vi "Speed from Pulse Position (No State).vi"(6 "state in":T1, 7 "Blocks/Pulse":dbl, 10 "pulse/revolution (1)":dbl, 11 "speed position info":T2) -> (3 "CPS":dbl, 4 "state out":T1)   [LabVIEW 2012, in "Measurement Channels.lvlib" / "Tachometer.lvclass"]
uses:
  Tachometer.lvclass
  <vilib>/addons/Sound and Vibration/Order Analysis/Misc/OAT Position Info.ctl
  <vilib>/Analysis/baseanly.llb/Mean (DBL).vi
  <vilib>/Analysis/NI_AALBase.lvlib
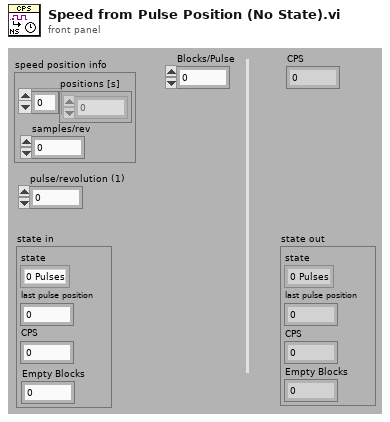
[diagram p1: front panel]
types:
  T1 = cluster{"state":enum16{"0 Pulses", "1 Pulse", "2+ Pulses"}, "last pulse position":dbl, "CPS":dbl, "Empty Blocks":i32}
  T2 = typedef "OAT Position Info.ctl" = cluster{"positions [s]":dbl[], "samples/rev":dbl}
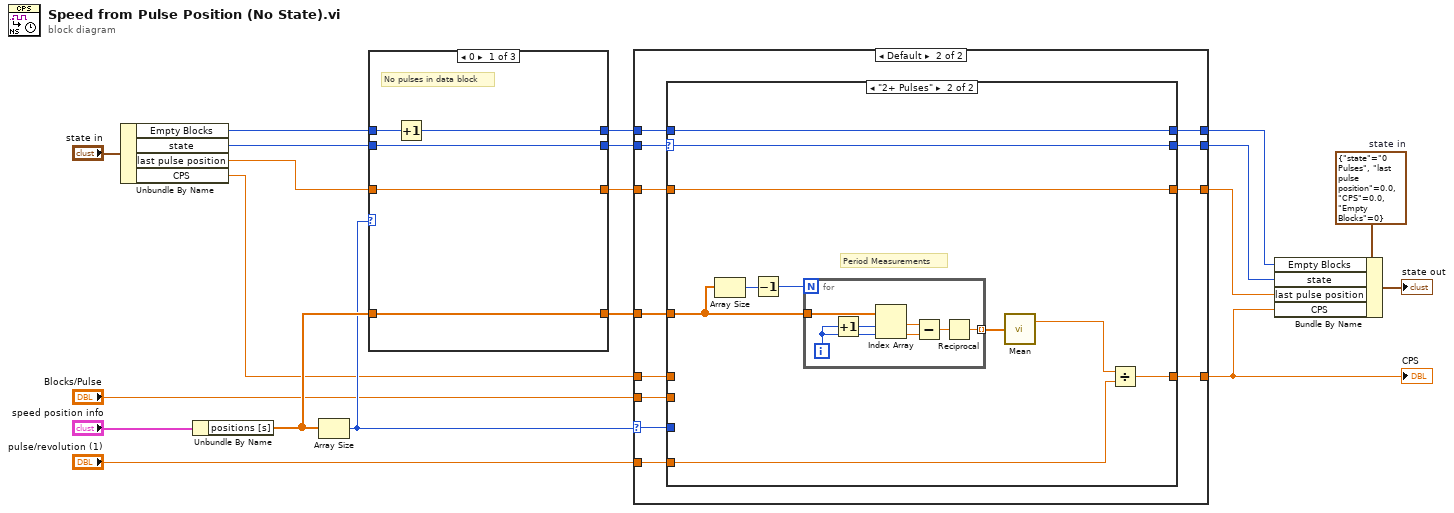
[diagram p0: block diagram]
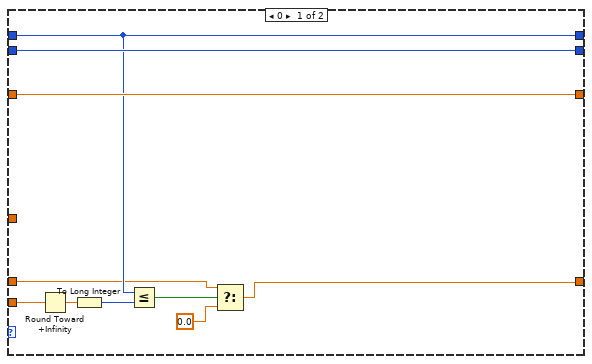
[diagram p2: hidden frame]
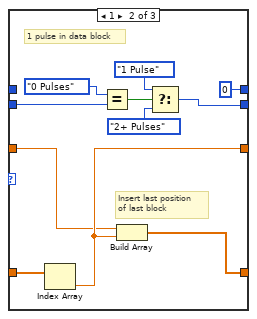
[diagram p4: hidden frame]
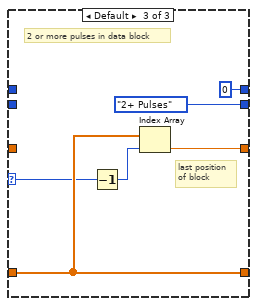
[diagram p5: hidden frame]
diagram:
  w6 = T1 {"state"=enum."0 Pulses", "last pulse position"=0.0, "CPS"=0.0, "Empty Blocks"=0}  # state in
  n1 = Unbundle By Name("state in") -> ("Empty Blocks"=w4:i32, "state"=w9:enum16{"0 Pulses", "1 Pulse", "2+ Pulses"}, "last pulse position"=w8:dbl, "CPS"=w7:dbl)
  n2 = Unbundle By Name("speed position info") -> ("positions [s]"=w16:dbl[])
  n3 = Array Size(array=w16) -> (size(s)=w14:i32)
  n4 = case shown="0" w14 {
    selector: w14 -> [_ _ w41]
    tunnel: w8 -> [w24 w33 _]
    tunnel: [w24 w34 w39] -> w13
    tunnel: w9 -> [w25 w31 _]
    tunnel: [w25 w27 enum16{"0 Pulses", "1 Pulse", "2+ Pulses"}."2+ Pulses" ("Enum")] -> w11
    tunnel: w16 -> [w23 w36 w42]
    tunnel: [w23 w35 w42] -> w10
    tunnel: w4 -> [w22 _ _]
    tunnel: [w21 0 0] -> w3
    frame 0 {
      # "No pulses in data block"
      n5 = Increment(x=w22) -> (x+1=w21:i32)
    }
    frame 1 {
      # "Insert last position\nof last block"
      # "1 pulse in data block"
      n6 = Index Array(array=w36) -> (element=w34:dbl)  [unwired: 1 in]
      n7 = Equal?(x=enum16{"0 Pulses", "1 Pulse", "2+ Pulses"}."0 Pulses" ("Enum"), y=w31) -> (x = y?=w30:bool)
      n8 = Build Array(w33, w34) -> (w35:dbl[])
      n9 = Select(t=enum16{"0 Pulses", "1 Pulse", "2+ Pulses"}."1 Pulse" ("Enum"), s=w30, f=enum16{"0 Pulses", "1 Pulse", "2+ Pulses"}."2+ Pulses" ("Enum")) -> (s? t:f=w27:enum16{"0 Pulses", "1 Pulse", "2+ Pulses"})
    }
    frame Default {
      # "last position\nof block"
      # "2 or more pulses in data block"
      n10 = Decrement(x=w41) -> (x-1=w40:i32)
      n11 = Index Array(array=w42, index=w40) -> (element=w39:dbl)
    }
  }
  n12 = case shown="Default" w14 {
    selector: w14 -> [_ w56]
    tunnel: w10 -> [_ w64]
    tunnel: w11 -> [w52 w63]
    tunnel: [w43 w62] -> w20
    tunnel: w7 -> [w44 w61]
    tunnel: "pulse/revolution (1)" -> [_ w60]
    tunnel: [w52 w59] -> w17
    tunnel: w13 -> [w51 w58]
    tunnel: [w51 w57] -> w18
    tunnel: w3 -> [w45 w55]
    tunnel: [w45 w54] -> w2
    tunnel: "Blocks/Pulse" -> [w46 w53]
    frame 0 {
      n13 = Round Toward +Infinity(x=w46) -> (ceil(x): smallest int >= x=w50:dbl)
      n14 = To Long Integer(number=w50) -> (32bit integer=w47:i32)
      n15 = Less Or Equal?(x=w45, y=w47) -> (x <= y?=w49:bool)
      n16 = Select(t=w44, s=w49, f=0.0) -> (s? t:f=w43:dbl)
    }
    frame Default {
      n17 = case shown="\"2+ Pulses\"" w63 {
        selector: w63 -> [w68 w71]
        tunnel: [w65 w78] -> w62
        tunnel: w64 -> [_ w77]
        tunnel: w61 -> [w65 _]
        tunnel: w60 -> [_ w76]
        tunnel: w56 -> [_ _]
        tunnel: [w68 w71] -> w59
        tunnel: w58 -> [w67 w72]
        tunnel: [w67 w72] -> w57
        tunnel: w55 -> [w66 w70]
        tunnel: [w66 w70] -> w54
        tunnel: w53 -> [_ _]
        frame "0 Pulses", "1 Pulse" {
        }
        frame "2+ Pulses" {
          # "Period Measurements"
          n18 = Array Size(array=w77) -> (size(s)=w75:i32)
          n19 = Decrement(x=w75) -> (x-1=w73:i32)
          n20 = for {
            N: w73 -> [_]
            tunnel: w77 -> [w85]
            tunnel: [w84] -> w74 mode=indexing
            i -> [w80]
            n21 = Increment(x=w80) -> (x+1=w81:i32)
            n22 = Index Array(array=w85, index #1=w81, index #2=w80) -> (element #1=w79:dbl, element #2=w82:dbl)
            n23 = Subtract(x=w79, y=w82) -> (x-y=w83:dbl)
            n24 = Reciprocal(x=w83) -> (1/x=w84:dbl)
          }
          n25 = call-poly <vilib>:"Mean.vi"("X"=w74) -> ("mean"=w69:dbl)  [unwired: 1 out]
          n26 = Divide(x=w69, y=w76) -> (x/y=w78:dbl)
        }
      }
    }
  }
  "CPS" <- w20
  n27 = Bundle By Name(cluster=w6, "Empty Blocks"=w2, "state"=w17, "last pulse position"=w18, "CPS"=w20) -> (→"state out":T1)
